vi "Calibrate_Decision.vi"(8 "error in (no error)":errorcluster, 10 "reference":refnum<vi>) -> (0 "error out":errorcluster)   [LabVIEW 2020]
doc: "Use this template to build a VI to use as a subVI."
panel:
  in  "End":bool
  in  "Retest":bool
  # "Serial Poll Byte Check Failed!"
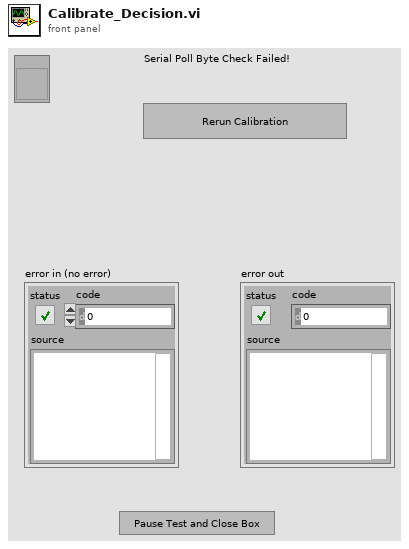
[diagram p1: front panel]
types:
  T1 = enum32{"Invalid", "Standard", "Closed", "Hidden", "Minimized", "Maximized"}
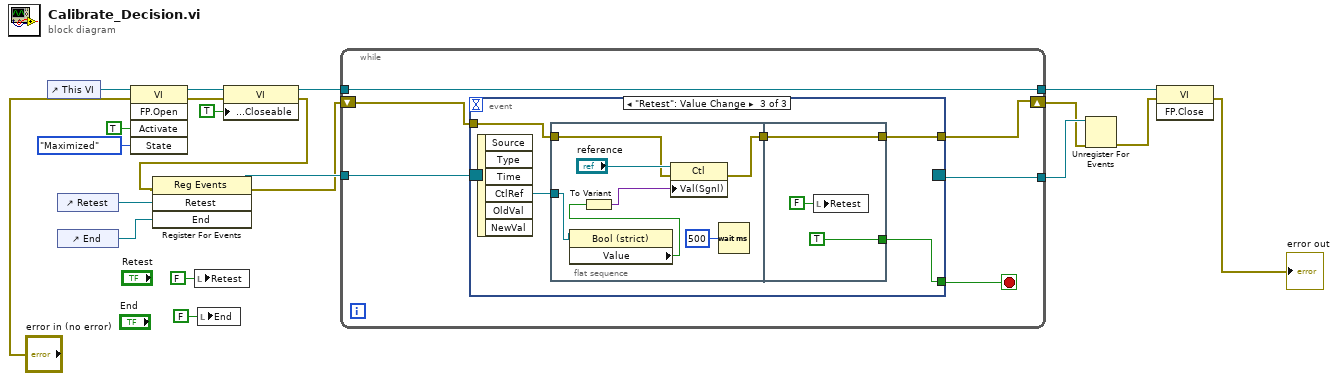
[diagram p0: block diagram]
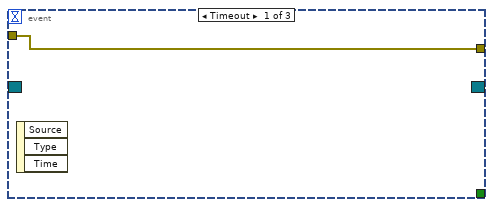
[diagram p2: hidden frame]
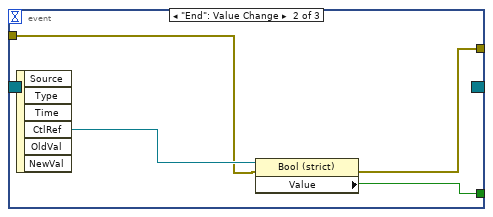
[diagram p3: hidden frame]
diagram:
  n1 = control-ref of="This VI"() -> (w20:refnum<vi>)
  n2 = control-ref of="Retest"() -> (w9:refnum<vi>)
  n3 = control-ref of="End"() -> (w8:refnum<vi>)
  n4 = invoke class="VI" method="FP.Open"(reference=w20, error in="error in (no error)", "Activate"=TRUE ("Activate?"), "State"=T1."Maximized") -> (reference out=w18:refnum<vi>, error out=w13:errorcluster)  [unwired: 1 in, 3 out]
  n5 = local write "Retest"(FALSE ("Retest")) -> ()
  n6 = local write "End"(FALSE ("End")) -> ()
  n7 = property class="VI"(reference=w18, error in=w13, "Front Panel.Closeable"=TRUE ("Front Panel Window:Closeable")) -> (reference out=w17:refnum<vi>, error out=w5:errorcluster)
  n8 = register-events(error in=w5, w9, w8) -> (reference out=w10:refnum<event-registration>, error out=w4:errorcluster)  [unwired: 1 in]
  n9 = while {
    tunnel: w17 -> [w25]
    tunnel: [w25] -> w19
    tunnel: w10 -> [w24]
    shift-right: [w22] -> w2
    shift-left: w4 -> [w23]
    tunnel: [w21] -> w3
    stop <- w26 stop-if-true
    n10 = event shown="[2] \"Retest\": Value Change" {
      selector: w24 -> [_ _ _]
      dyn-events: [_ _ _] -> w21
      timeout: _ -> [_ _ _]
      tunnel: [_ w30 w35] -> w26
      tunnel: w23 -> [w27 w29 w34]
      tunnel: [w27 w28 w33] -> w22
      event Timeout {
        n11 = event-data() -> ()  [unwired: 1 in, 3 out]
      }
      event "End": Value Change {
        n12 = event-data() -> ("CtlRef"=w31:refnum<vi>)  [unwired: 1 in, 5 out]
        n13 = property class="Bool (strict)"(reference=w31, error in=w29) -> (error out=w28:errorcluster, "Value"=w30:bool)  [unwired: 1 out]
      }
      event "Retest": Value Change {
        n14 = event-data() -> ("CtlRef"=w36:refnum<vi>)  [unwired: 1 in, 5 out]
        n15 = flat-sequence {
          tunnel: w36 -> [w40]
          tunnel: w34 -> [w38]
          tunnel: [w37] -> w32
          tunnel: [TRUE ("End")] -> w35
          tunnel: [w44] -> w33
          tunnel: w32 -> [w44]
          frame #0 {
            n16 = property class="Bool (strict)"(reference=w40) -> ("Value"=w41:bool)  [unwired: 1 in, 2 out]
            n17 = To Variant(anything=w41) -> (Variant=w42:variant)
            n18 = property class="Ctl"(reference="reference", error in=w38, "Val(Sgnl)"=w42) -> (error out=w37:errorcluster)  [unwired: 1 out]
            n19 = Wait (ms)(milliseconds to wait=u32 500) -> ()  [unwired: 1 out]
          }
          frame #1 {
            n20 = local write "Retest"(FALSE ("Retest")) -> ()
          }
        }
      }
    }
  }
  n21 = Unregister For Events(event registration refnum=w3, error in=w2) -> (error out=w1:errorcluster)
  n22 = invoke class="VI" method="FP.Close"(reference=w19, error in=w1) -> (error out=→"error out":errorcluster)  [unwired: 1 in, 2 out]
